vi "Callback.vi"(8 "error in (no error)":errorcluster, 9 "Message Data":variant, 10 "Message":string, 11 "Synchronous Request Callback in":refnum<class "Synchronous Request Callback.lvclass">) -> (0 "error out":errorcluster)   [LabVIEW 2020, in "Synchronous Request Callback.lvclass"]
uses:
  Synchronous Request Callback.lvclass
  Process/Protected/Messaging/Response Message Cluster.ctl
  Synchronous Request Callback.lvclass/Synchronous Request Callback.ctl
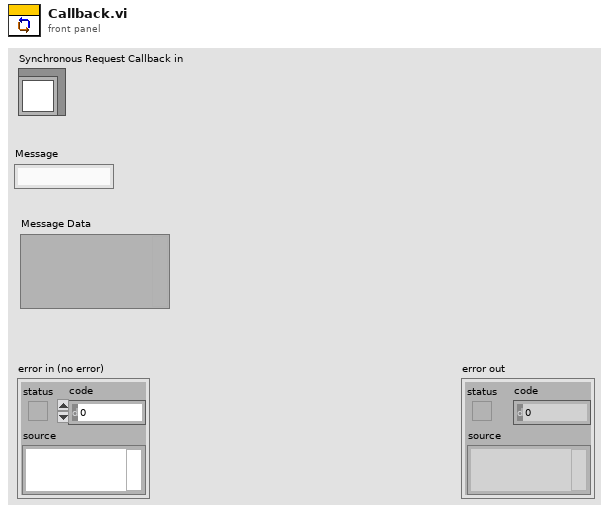
[diagram p1: front panel]
types:
  T1 = typedef "Synchronous Request Callback.lvclass/Response Message Cluster.ctl" = cluster{"Message":string, "Message Data":variant, "Error Out":errorcluster}
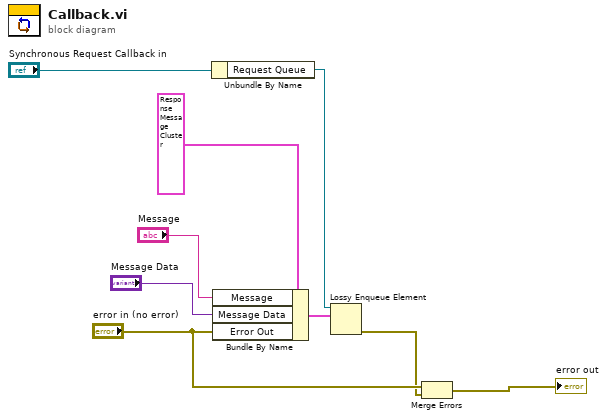
[diagram p0: block diagram]
diagram:
  n1 = Unbundle By Name("Synchronous Request Callback in") -> ("Request Queue"=w1:refnum<queue>)
  n2 = Bundle By Name(cluster=T1 {"Message"="", "Message Data"=variant, "Error Out"={"status"=FALSE, "code"=0, "source"=""}} ("notification"), "Message"="Message", "Message Data"="Message Data", "Error Out"="error in (no error)") -> (w7:T1)
  n3 = Lossy Enqueue Element(queue=w1, element=w7) -> (error out=w2:errorcluster)  [unwired: 1 in, 3 out]
  n4 = Merge Errors("error in (no error)", w2) -> (→"error out":errorcluster)
